vi "VsEP-Parse Data.vi"(0 "Runtime":T1, 1 "Reject OverRide":bool, 2 "Rej Thresh µV":dbl=15.0, 5 "Data":dbl[](array[numeric]), 7 "scale factor":dbl=1.0, 9 "Acquired In":i32, 11 "error in (no error)":errorcluster) -> (3 "Finished?":bool, 4 "Frej":dbl, 6 "RunSum1":dbl[](array[numeric]), 8 "RunSum2":dbl[](array[numeric]), 10 "Acquired Out":i32, 14 "Ntries":i32, 15 "error out":errorcluster)   [LabVIEW 2020]
uses:
  Typedefs/VsEP-Runtime Data.ctl
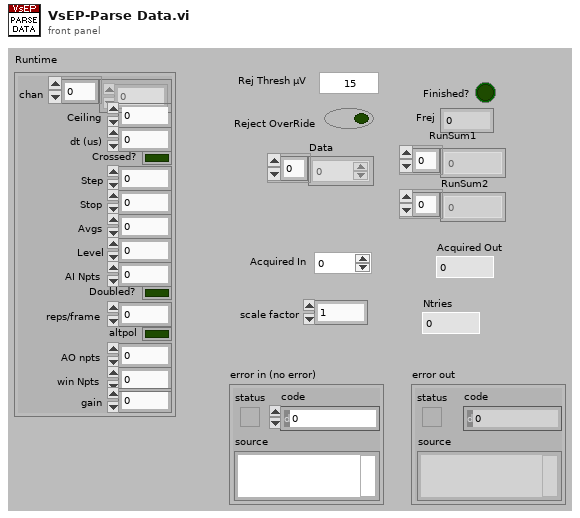
[diagram p1: front panel]
types:
  T1 = typedef "VsEP-Runtime Data.ctl" = cluster{"chan":i32[], "Ceiling":dbl, "dt (us)":dbl, "Crossed?":bool, "Step":dbl, "Stop":i32, "Avgs":i32, "Level":dbl, "AI Npts":i32, "Doubled?":bool, "reps/frame":i32, "altpol":bool, "AO npts":i32, "win Npts":i32, "gain":dbl}
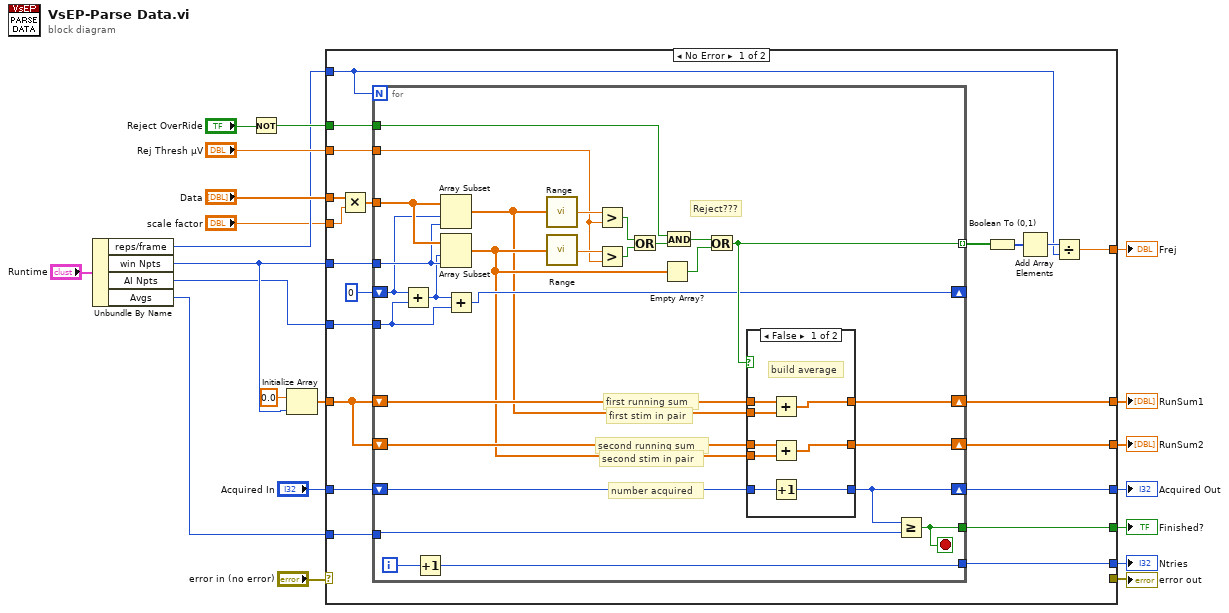
[diagram p0: block diagram]
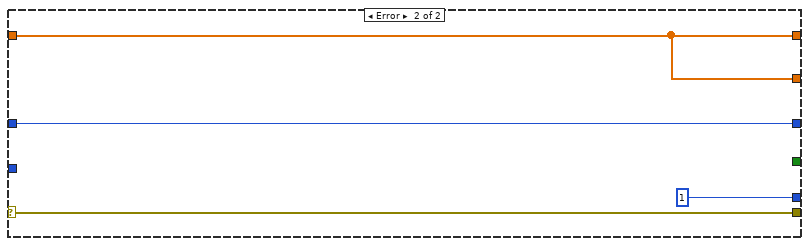
[diagram p3: hidden frame]
diagram:
  n1 = Unbundle By Name("Runtime") -> ("reps/frame"=w5:i32, "win Npts"=w9:i32, "AI Npts"=w1:i32, "Avgs"=w8:i32)
  n2 = Not(x="Reject OverRide") -> (.not. x?=w17:bool)
  n3 = Initialize Array(0.0 ("element"), w9) -> (w13:dbl[])
  n4 = case shown="No Error" "error in (no error)" {
    selector: "error in (no error)" -> [_ w85]
    tunnel: [_ w85] -> w20
    tunnel: "Data" -> [w42 _]
    tunnel: w17 -> [w41 _]
    tunnel: "Rej Thresh µV" -> [w40 _]
    tunnel: w9 -> [w39 _]
    tunnel: w5 -> [w23 _]
    tunnel: w1 -> [w38 _]
    tunnel: [w22 _] -> w14
    tunnel: w13 -> [w37 w83]
    tunnel: [w35 w83] -> w2
    tunnel: [w34 w83] -> w3
    tunnel: [w33 w84] -> w12
    tunnel: "Acquired In" -> [w32 w84]
    tunnel: w8 -> [w31 _]
    tunnel: [w30 _] -> w7
    tunnel: [w29 1] -> w6
    tunnel: "scale factor" -> [w27 _]
    frame No Error {
      n5 = Multiply(x=w42, y=w27) -> (x*y=w28:dbl[])
      n6 = for {
        N: w23 -> [_]
        tunnel: w28 -> [w63]
        tunnel: w41 -> [w62]
        tunnel: w40 -> [w61]
        tunnel: w39 -> [w60]
        tunnel: w38 -> [w51]
        tunnel: [w59] -> w24 mode=indexing
        shift-right: [w49] -> w33
        shift-left: w32 -> [w58]
        shift-right: [w56] -> w35
        shift-left: w37 -> [w57]
        shift-right: [w55] -> w34
        shift-left: w37 -> [w54]
        shift-right: [w50] -> _
        shift-left: 0 -> [w53]
        tunnel: w31 -> [w48]
        tunnel: [w47] -> w30
        tunnel: [w45] -> w29
        i -> [w46]
        stop <- w47 stop-if-true
        # "Reject???"
        # "second running sum"
        # "first running sum"
        # "second stim in pair"
        # "first stim in pair"
        # "number acquired"
        n7 = Add(x=w53, y=w51) -> (x+y=w52:i32)
        n8 = Increment(x=w46) -> (x+1=w45:i32)
        n9 = Array Subset(array=w63, index=w53, length=w60) -> (w43:dbl[])
        n10 = Array Subset(array=w63, index=w52, length=w60) -> (w44:dbl[])
        n11 = Add(x=w52, y=w51) -> (x+y=w50:i32)
        n12 = call "Range.vi"("Array"=w43) -> ("Range"=w65:dbl)
        n13 = call "Range.vi"("Array"=w44) -> ("Range"=w64:dbl)
        n14 = Greater?(x=w65, y=w61) -> (0:w67:bool)
        n15 = Greater?(x=w64, y=w61) -> (0:w66:bool)
        n16 = Or(x=w67, y=w66) -> (x .or. y?=w68:bool)
        n17 = Empty Array?(array=w44) -> (empty?=w69:bool)
        n18 = And(x=w62, y=w68) -> (x .and. y?=w70:bool)
        n19 = Or(x=w70, y=w69) -> (x .or. y?=w59:bool)
        n20 = case shown="False" w59 {
          tunnel: w43 -> [w76 _]
          tunnel: w44 -> [w72 _]
          tunnel: w58 -> [w78 w81]
          tunnel: [w77 w81] -> w49
          tunnel: w57 -> [w75 w80]
          tunnel: [w74 w80] -> w56
          tunnel: [w73 w79] -> w55
          tunnel: w54 -> [w71 w79]
          frame False {
            # "build average"
            n21 = Add(x=w75, y=w76) -> (x+y=w74:dbl[])
            n22 = Add(x=w71, y=w72) -> (x+y=w73:dbl[])
            n23 = Increment(x=w78) -> (x+1=w77:i32)
          }
          frame True {
          }
        }
        n24 = Greater Or Equal?(x=w49, y=w48) -> (x >= y?=w47:bool)
      }
      n25 = Boolean To (0,1)(Boolean=w24) -> (0, 1=w26:i16[])
      n26 = Add Array Elements(numeric array=w26) -> (sum=w25:i16)
      n27 = Divide(x=w25, y=w23) -> (x/y=w22:dbl)
    }
    frame Error {
    }
  }
  "error out" <- w20
  "Frej" <- w14
  "RunSum1" <- w2
  "RunSum2" <- w3
  "Acquired Out" <- w12
  "Finished?" <- w7
  "Ntries" <- w6
